vi "Set Front Panel Panel Size.vi"(8 "error in":errorcluster, 10 "Panel Bounds":T1, 11 "VI Ref":refnum<vi>) -> (0 "error out":errorcluster, 3 "VI Ref":refnum<vi>)   [LabVIEW 2014]
doc: "Makes FP resizable and sets FP bounds."
uses:
  <vilib>/Utility/miscctls.llb/LVRectTypeDef.ctl
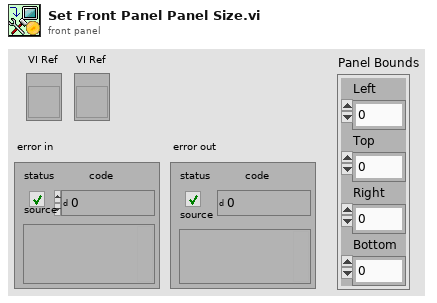
[diagram p1: front panel]
types:
  T1 = typedef "LVRectTypeDef.ctl" = cluster{"Left":i16, "Top":i16, "Right":i16, "Bottom":i16}
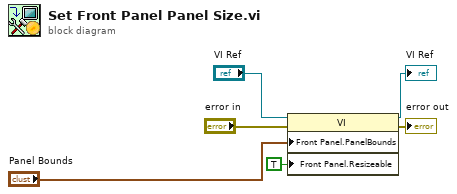
[diagram p0: block diagram]
diagram:
  n1 = property class="VI"(reference="VI Ref", error in="error in", "Front Panel.PanelBounds"="Panel Bounds", "Front Panel.Resizeable"=TRUE ("Front Panel Window:Resizable")) -> (reference out=→"VI Ref":refnum<vi>, error out=→"error out":errorcluster)
